vi "gamma_correction_array_float.vi"(8 "i32_ar_first_and_last_pixel":i32[][](array[numeric]), 11 "adapted image px array":dbl[][][](array[numeric])) -> (3 "i16_normalized unwrapped array":dbl[][][](array[numeric]))   [LabVIEW 2011]
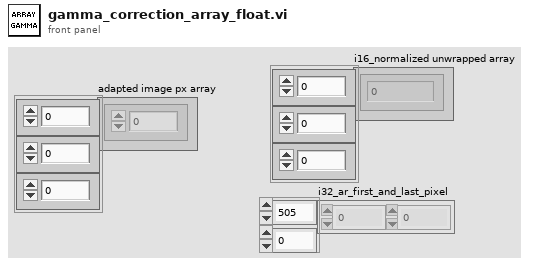
[diagram p1: front panel]
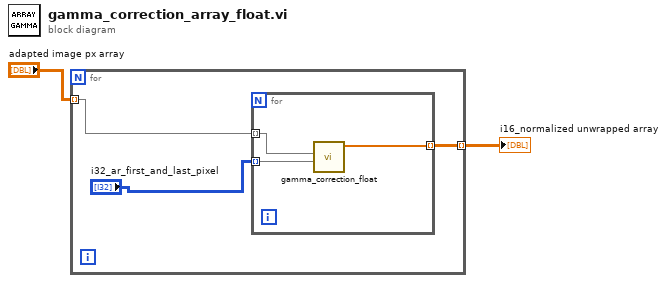
[diagram p0: block diagram]
diagram:
  n1 = for {
    tunnel: "adapted image px array" -> [w5] mode=indexing
    tunnel: [w4] -> w1 mode=indexing
    n2 = for {
      tunnel: w5 -> [w8] mode=indexing
      tunnel: "i32_ar_first_and_last_pixel" -> [w7] mode=indexing
      tunnel: [w6] -> w4 mode=indexing
      n3 = call "gamma_correction_float.vi"("i32_ar_first_and_last_pixel"=w7, "u8_pxar_dist"=w8) -> ("i16_normalized unwrapped array"=w6:dbl[])  [unwired: 9 in]
    }
  }
  "i16_normalized unwrapped array" <- w1
